vi "Inc_Dec Frequency.vi"() -> (0 "Freq (Hz)":dbl[](array[numeric])=[2.0, 3.0, 4.0, 6.0, 8.0, 10.0, 12.0, 14.0, 16.0, 18.0, 20.0, 22.0, 24.0, 26.0, 28.0, 30.0, 35.0, 40.0, 45.0, 50.0, 55.0, 60.0, 65.0, 70.0, 75.0, 80.0, 85.0, 90.0, 95.0, 100.0, 110.0, 120.0, 130.0, 140.0, 150.0, 160.0, 170.0, 180.0, 190.0, 200.0, 225.0, 250.0, 275.0, 300.0, 325.0, 350.0, 375.0, 400.0, 500.0, 600.0, 700.0, 800.0, 900.0, 1000.0, 1100.0, 1200.0, 1300.0, 1400.0, 1500.0, 1600.0, 1700.0, 1800.0, 1900.0, 2000.0])   [LabVIEW 2010]
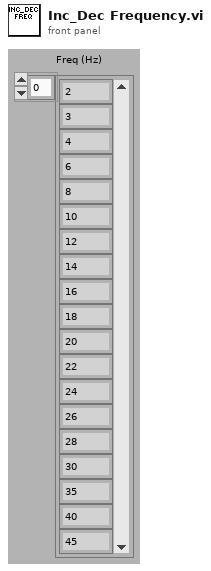
[diagram p1: front panel]
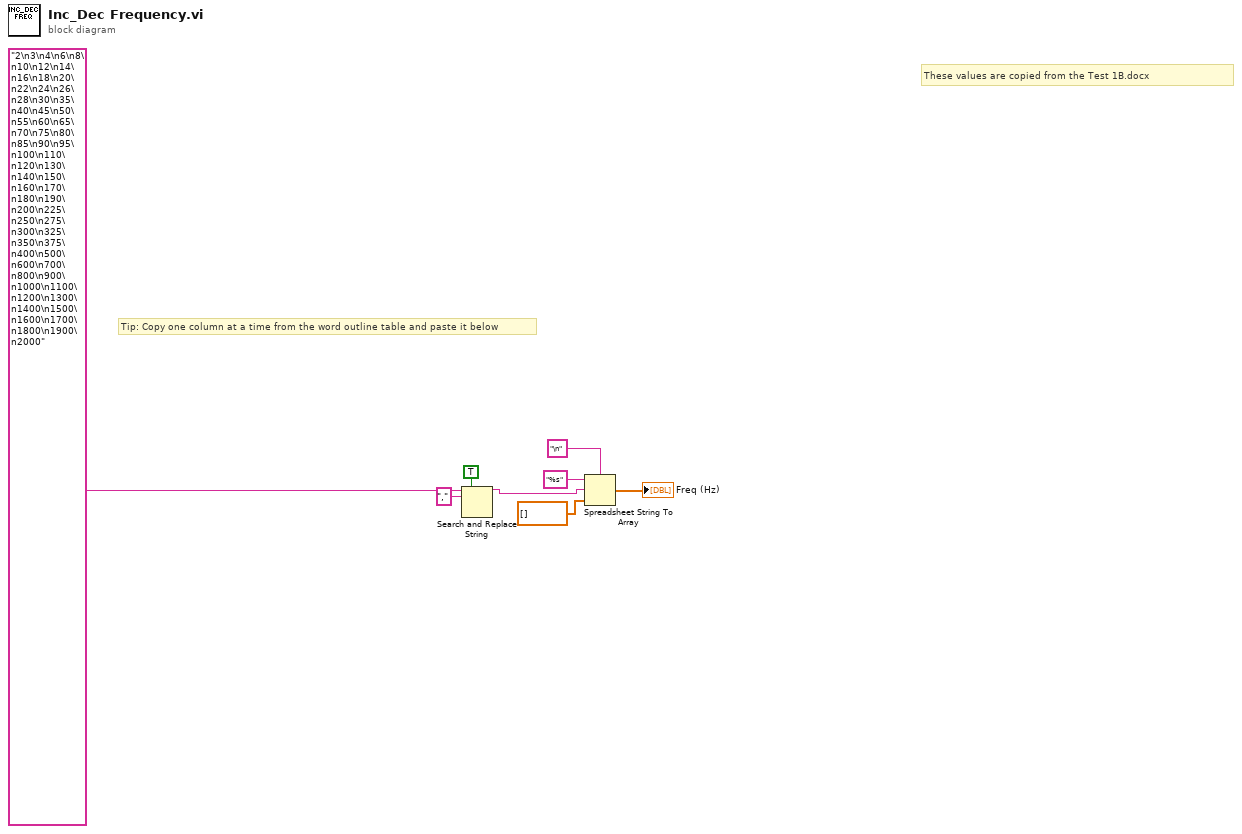
[diagram p0: block diagram]
diagram:
  # "Tip: Copy one column at a time from the word outline table and paste it below"
  # "These values are copied from the Test 1B.docx"
  n1 = Search and Replace String(replace all?=TRUE ("replace all? (F)"), input string="2\n3\n4\n6\n8\n10\n12\n14\n16\n18\n20\n22\n24\n26\n28\n30\n35\n40\n45\n50\n55\n60\n65\n70\n75\n80\n85\n90\n95\n100\n110\n120\n130\n140\n150\n160\n170\n180\n190\n200\n225\n250\n275\n300\n325\n350\n375\n400\n500\n600\n700\n800\n900\n1000\n1100\n1200\n1300\n1400\n1500\n1600\n1700\n1800\n1900\n2000" ("Pulse 1"), search string=",") -> (result string=w4:string)  [unwired: 5 in, 3 out]
  n2 = Spreadsheet String To Array(delimiter (Tab)="\n", format string="%s", spreadsheet string=w4, array type (2D Dbl)=dbl[] []) -> (array=→"Freq (Hz)":dbl[])
